vi "Using JSON for files.vi"() -> ()   [LabVIEW 2025, in "IT-M3900C.lvlib"]
uses:
  IT-M3900C.lvlib
panel:
  out "Voltage Level":dbl[](array[numeric])
  out "value":T1
  in  "Test Settings":T1
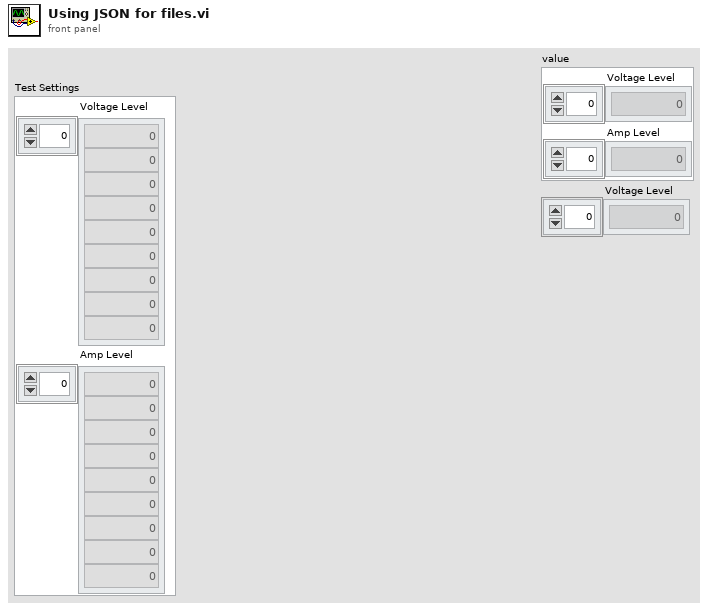
[diagram p1: front panel]
types:
  T1 = cluster{"Voltage Level":dbl[], "Amp Level":dbl[]}
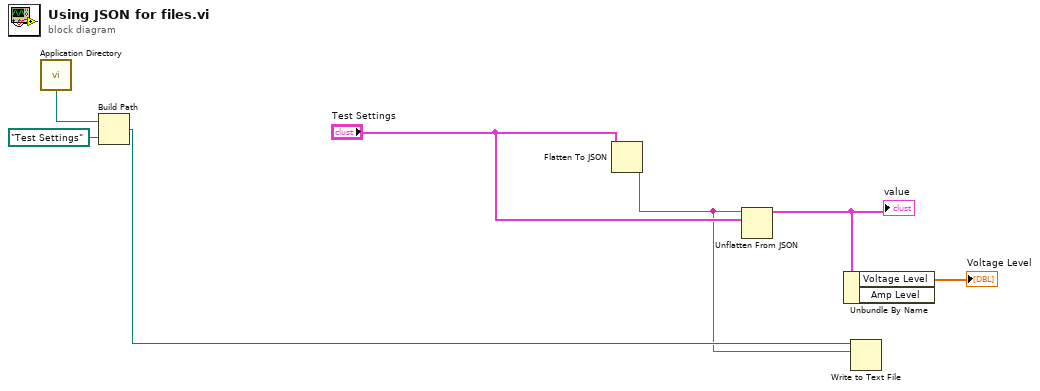
[diagram p0: block diagram]
diagram:
  n1 = call <vilib>:"Application Directory.vi"() -> ("Application Directory"=w7:path)
  n2 = Build Path(base path=w7, name or relative path=path "Test Settings") -> (appended path=w3:path)
  n3 = Flatten To JSON(anything="Test Settings") -> (JSON string=w1:string)  [unwired: 2 in, 1 out]
  n4 = Unflatten From JSON(JSON string=w1, type and defaults="Test Settings") -> (value=w2:T1)  [unwired: 5 in, 1 out]
  "value" <- w2
  n5 = Unbundle By Name(w2) -> ("Voltage Level"=→"Voltage Level":dbl[])  [unwired: 1 out]
  n6 = Write to Text File(file (use dialog)=w3, text=w1) -> ()  [unwired: 2 in, 3 out]
